vi "Prueba_velocidad_servo.vi"() -> ()   [LabVIEW 2020]
panel:
  out "Velocidad RPM":dbl(knob) scale=0.0..2000.0
  in  "Control de Velocidad RPM":dbl(knob) scale=0.0..2000.0 scale format="%#_5g"
  out "ON/OFF":bool[](array[boolean])
  in  "Enable":bool[](array[boolean])
  in  "?":bool
  # "Control Servo"
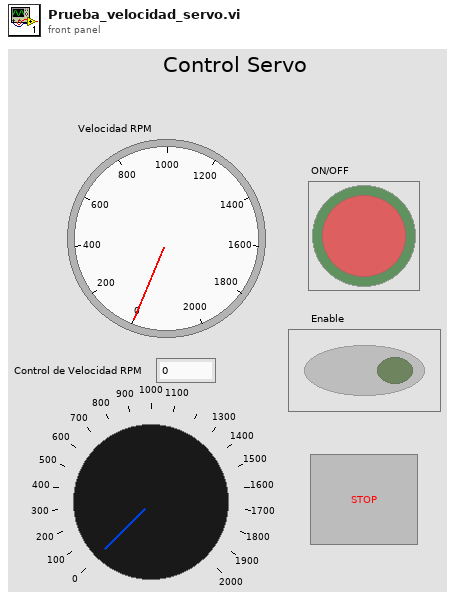
[diagram p1: front panel]
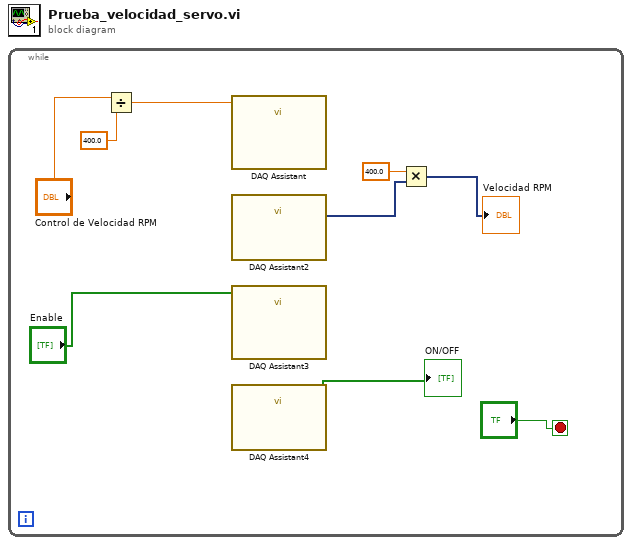
[diagram p0: block diagram]
diagram:
  n1 = while {
    stop <- "?" stop-if-true
    n2 = Divide(x="Control de Velocidad RPM", y=400.0 ("x")) -> (x/y=w6:dbl)
    n3 = call "DAQ Assistant"("data"=w6) -> ()  [unwired: 17 in, 2 out]
    n4 = call "DAQ Assistant2"() -> ("data"=w4:dynamicdata)  [unwired: 17 in, 2 out]
    n5 = call "DAQ Assistant3"("data"="Enable") -> ()  [unwired: 17 in, 2 out]
    n6 = call "DAQ Assistant4"() -> ("data"=→"ON/OFF":bool[])  [unwired: 17 in, 2 out]
    n7 = Multiply(x=400.0, y=w4) -> (x*y=→"Velocidad RPM":dynamicdata)
  }
